vi "Set Mono Prop.vi"(8 "error in (no error)":errorcluster, 9 "Current Wavelength":dbl[unit], 10 "Current Grating":u16(ring) items=["1200 gr/mm"=1200, "600 gr/mm"=600], 11 "IJYCCDReqd In":refnum<k7>) -> (0 "error out":errorcluster, 3 "IJYCCDReqd out":refnum<k7>)   [LabVIEW 2015]
doc: "Sets the TRIAX 550 Mono properties in the CCD object. Call the Wavelength Coverage method for spectrum wavlength coverage."
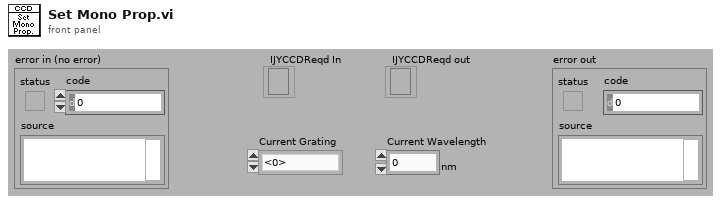
[diagram p1: front panel]
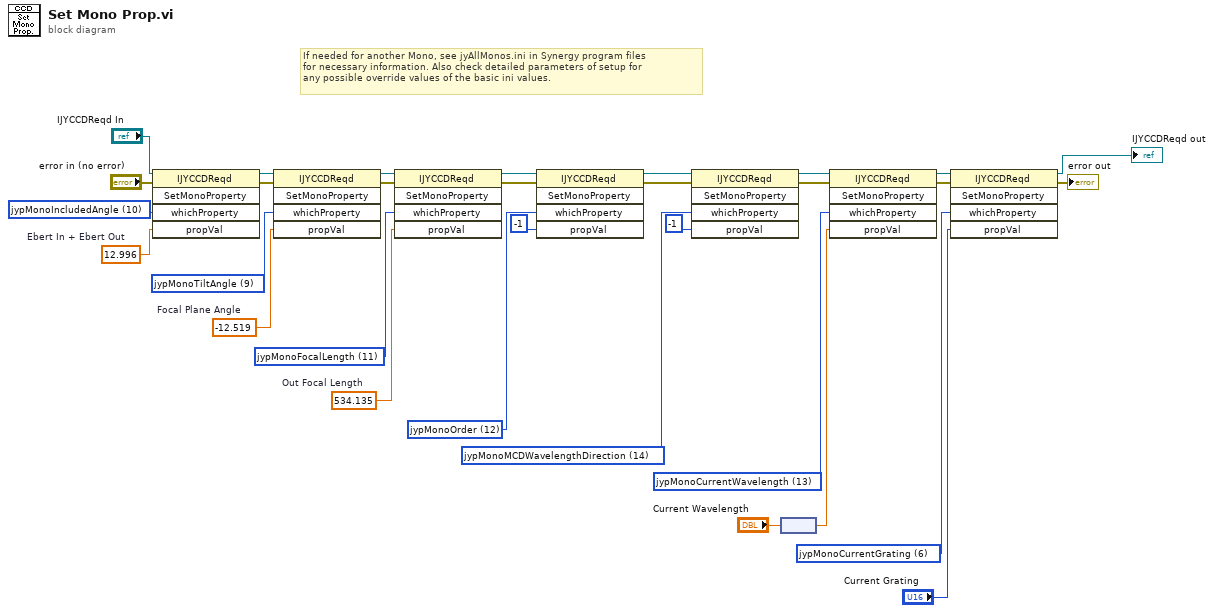
[diagram p0: block diagram]
diagram:
  w6 = 534.135  # Out Focal Length
  w7 = -12.519  # Focal Plane Angle
  w8 = 12.996  # Ebert In + Ebert Out
  w24 = 13 items=["jyUndefined", "jypMonoLinearDispersion", "jypMonoBacklashAmount", "jypMonoStepsPerUnit", "jypMonoBaseUnits", "jypMonoBaseGrating", "jypMonoCurrentGrating", "jypMonoMaxLimit", "jypMonoMinLimit", "jypMonoTiltAngle", "jypMonoIncludedAngle", "jypMonoFocalLength", "jypMonoOrder", "jypMonoCurrentWavelength", "jypMonoMCDWavelengthDirection", "jypBandpassUnits", "jypSlitMaxLimit", "jypSlitMinLimit", "jypSlitBackLashAmount", "jypSlitBaseUnits", "jypSlitStepsPerUnit", "jypLaserLine", "jypTotalHardwarePropertiesPlusOne", "jypCurrentTurretPosition"] ("whichProperty")
  w25 = 14 items=["jyUndefined", "jypMonoLinearDispersion", "jypMonoBacklashAmount", "jypMonoStepsPerUnit", "jypMonoBaseUnits", "jypMonoBaseGrating", "jypMonoCurrentGrating", "jypMonoMaxLimit", "jypMonoMinLimit", "jypMonoTiltAngle", "jypMonoIncludedAngle", "jypMonoFocalLength", "jypMonoOrder", "jypMonoCurrentWavelength", "jypMonoMCDWavelengthDirection", "jypBandpassUnits", "jypSlitMaxLimit", "jypSlitMinLimit", "jypSlitBackLashAmount", "jypSlitBaseUnits", "jypSlitStepsPerUnit", "jypLaserLine", "jypTotalHardwarePropertiesPlusOne", "jypCurrentTurretPosition"] ("whichProperty")
  w26 = 12 items=["jyUndefined", "jypMonoLinearDispersion", "jypMonoBacklashAmount", "jypMonoStepsPerUnit", "jypMonoBaseUnits", "jypMonoBaseGrating", "jypMonoCurrentGrating", "jypMonoMaxLimit", "jypMonoMinLimit", "jypMonoTiltAngle", "jypMonoIncludedAngle", "jypMonoFocalLength", "jypMonoOrder", "jypMonoCurrentWavelength", "jypMonoMCDWavelengthDirection", "jypBandpassUnits", "jypSlitMaxLimit", "jypSlitMinLimit", "jypSlitBackLashAmount", "jypSlitBaseUnits", "jypSlitStepsPerUnit", "jypLaserLine", "jypTotalHardwarePropertiesPlusOne", "jypCurrentTurretPosition"] ("whichProperty")
  w27 = 11 items=["jyUndefined", "jypMonoLinearDispersion", "jypMonoBacklashAmount", "jypMonoStepsPerUnit", "jypMonoBaseUnits", "jypMonoBaseGrating", "jypMonoCurrentGrating", "jypMonoMaxLimit", "jypMonoMinLimit", "jypMonoTiltAngle", "jypMonoIncludedAngle", "jypMonoFocalLength", "jypMonoOrder", "jypMonoCurrentWavelength", "jypMonoMCDWavelengthDirection", "jypBandpassUnits", "jypSlitMaxLimit", "jypSlitMinLimit", "jypSlitBackLashAmount", "jypSlitBaseUnits", "jypSlitStepsPerUnit", "jypLaserLine", "jypTotalHardwarePropertiesPlusOne", "jypCurrentTurretPosition"] ("whichProperty")
  w28 = 9 items=["jyUndefined", "jypMonoLinearDispersion", "jypMonoBacklashAmount", "jypMonoStepsPerUnit", "jypMonoBaseUnits", "jypMonoBaseGrating", "jypMonoCurrentGrating", "jypMonoMaxLimit", "jypMonoMinLimit", "jypMonoTiltAngle", "jypMonoIncludedAngle", "jypMonoFocalLength", "jypMonoOrder", "jypMonoCurrentWavelength", "jypMonoMCDWavelengthDirection", "jypBandpassUnits", "jypSlitMaxLimit", "jypSlitMinLimit", "jypSlitBackLashAmount", "jypSlitBaseUnits", "jypSlitStepsPerUnit", "jypLaserLine", "jypTotalHardwarePropertiesPlusOne", "jypCurrentTurretPosition"] ("whichProperty")
  w29 = 10 items=["jyUndefined", "jypMonoLinearDispersion", "jypMonoBacklashAmount", "jypMonoStepsPerUnit", "jypMonoBaseUnits", "jypMonoBaseGrating", "jypMonoCurrentGrating", "jypMonoMaxLimit", "jypMonoMinLimit", "jypMonoTiltAngle", "jypMonoIncludedAngle", "jypMonoFocalLength", "jypMonoOrder", "jypMonoCurrentWavelength", "jypMonoMCDWavelengthDirection", "jypBandpassUnits", "jypSlitMaxLimit", "jypSlitMinLimit", "jypSlitBackLashAmount", "jypSlitBaseUnits", "jypSlitStepsPerUnit", "jypLaserLine", "jypTotalHardwarePropertiesPlusOne", "jypCurrentTurretPosition"] ("whichProperty")
  w23 = 6 items=["jyUndefined", "jypMonoLinearDispersion", "jypMonoBacklashAmount", "jypMonoStepsPerUnit", "jypMonoBaseUnits", "jypMonoBaseGrating", "jypMonoCurrentGrating", "jypMonoMaxLimit", "jypMonoMinLimit", "jypMonoTiltAngle", "jypMonoIncludedAngle", "jypMonoFocalLength", "jypMonoOrder", "jypMonoCurrentWavelength", "jypMonoMCDWavelengthDirection", "jypBandpassUnits", "jypSlitMaxLimit", "jypSlitMinLimit", "jypSlitBackLashAmount", "jypSlitBaseUnits", "jypSlitStepsPerUnit", "jypLaserLine", "jypTotalHardwarePropertiesPlusOne", "jypCurrentTurretPosition"] ("whichProperty")
  # "If needed for another Mono, see jyAllMonos.ini in Synergy program files\nfor necessary information. Also check detailed parameters of setup for\nany possible override values of the basic ini values."
  n1 = invoke class="IJYCCDReqd" method="SetMonoProperty"(reference="IJYCCDReqd In", error in="error in (no error)", "whichProperty"=w29, "propVal"=w8) -> (reference out=w22:refnum<k7>, error out=w21:errorcluster)  [unwired: 1 in, 3 out]
  n2 = invoke class="IJYCCDReqd" method="SetMonoProperty"(reference=w22, error in=w21, "whichProperty"=w28, "propVal"=w7) -> (reference out=w20:refnum<k7>, error out=w19:errorcluster)  [unwired: 1 in, 3 out]
  n3 = invoke class="IJYCCDReqd" method="SetMonoProperty"(reference=w20, error in=w19, "whichProperty"=w27, "propVal"=w6) -> (reference out=w18:refnum<k7>, error out=w17:errorcluster)  [unwired: 1 in, 3 out]
  n4 = invoke class="IJYCCDReqd" method="SetMonoProperty"(reference=w18, error in=w17, "whichProperty"=w26, "propVal"=-1) -> (reference out=w16:refnum<k7>, error out=w15:errorcluster)  [unwired: 1 in, 3 out]
  n5 = invoke class="IJYCCDReqd" method="SetMonoProperty"(reference=w16, error in=w15, "whichProperty"=w25, "propVal"=-1) -> (reference out=w14:refnum<k7>, error out=w13:errorcluster)  [unwired: 1 in, 3 out]
  n6 = node("Current Wavelength") -> (w1:dbl)
  n7 = invoke class="IJYCCDReqd" method="SetMonoProperty"(reference=w14, error in=w13, "whichProperty"=w24, "propVal"=w1) -> (reference out=w12:refnum<k7>, error out=w11:errorcluster)  [unwired: 1 in, 3 out]
  n8 = invoke class="IJYCCDReqd" method="SetMonoProperty"(reference=w12, error in=w11, "whichProperty"=w23, "propVal"="Current Grating") -> (reference out=→"IJYCCDReqd out":refnum<k7>, error out=→"error out":errorcluster)  [unwired: 1 in, 3 out]
